vi "DAQ-InitDevice.vi"(0 "message":string="Error al inicializar DAQ", 1 "DAQ Parameters":T1) -> (2 "DAQ Device OUT":T2, 3 "Inicializo DAQ?":bool, 4 "task OUT":refnum<k21>)   [LabVIEW 2010]
uses:
  <vilib>/DAQmx/create/channels.llb/DAQmx Create Channel (AO-Voltage-Basic).vi
  <vilib>/DAQmx/configure/timing.llb/DAQmx Timing (Use Waveform).vi
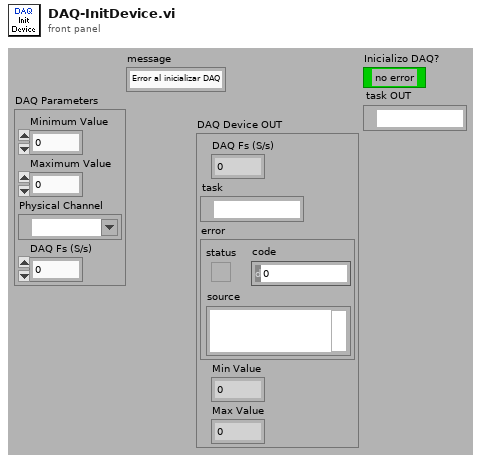
[diagram p1: front panel]
types:
  T1 = cluster{"Minimum Value":dbl, "Maximum Value":dbl, "Physical Channel":tag, "DAQ Fs (S/s)":dbl}
  T2 = cluster{"DAQ Fs (S/s)":dbl, "task":refnum<k21>, "error":errorcluster, "Min Value":dbl, "Max Value":dbl}
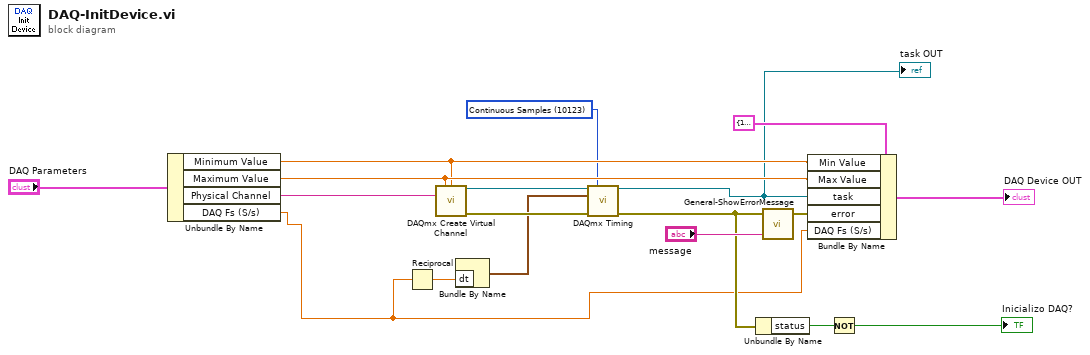
[diagram p0: block diagram]
diagram:
  w10 = 10123 items=["Finite Samples"=10178, "Continuous Samples"=10123, "Hardware Timed Single Point"=12522] ("sample mode")
  n1 = Unbundle By Name("DAQ Parameters") -> ("Minimum Value"=w15:dbl, "Maximum Value"=w16:dbl, "Physical Channel"=w13:tag, "DAQ Fs (S/s)"=w1:dbl)
  n2 = Reciprocal(x=w1) -> (1/x=w2:dbl)
  n3 = call-poly <vilib>:"DAQmx Create Virtual Channel.vi"("maximum value"=w16, "minimum value"=w15, "physical channels"=w13) -> ("task out"=w11:refnum<k21>, "error out"=w12:errorcluster)  [unwired: 11 in]
  n4 = Bundle By Name("dt"=w2) -> (w3:waveform(dbl))  [unwired: 1 in]
  n5 = call-poly <vilib>:"DAQmx Timing.vi"("task/channels in"=w11, "sample mode"=w10, "waveform"=w3, "error in"=w12) -> ("task out"=w6:refnum<k21>, "error out"=w5:errorcluster)  [unwired: 10 in]
  "task OUT" <- w6
  n6 = Unbundle By Name(w5) -> ("status"=w4:bool)
  n7 = call "General-ShowErrorMessage.vi"("message"="message", "Error IN"=w5) -> ("Error OUT"=w9:errorcluster)  [unwired: 3 in]
  n8 = Bundle By Name(cluster=T2 {"DAQ Fs (S/s)"=10000.0, "task"="", "error"={"status"=FALSE, "code"=0, "source"=""}, "Min Value"=-10.0, "Max Value"=10.0} ("DAQ Device IN"), "Min Value"=w15, "Max Value"=w16, "task"=w6, "error"=w9, "DAQ Fs (S/s)"=w1) -> (→"DAQ Device OUT":T2)
  n9 = Not(x=w4) -> (.not. x?=→"Inicializo DAQ?":bool)
